vi "Initialize.vi"(8 "error in (no error)":errorcluster) -> (0 "error out":errorcluster, 3 "config":T1={"Common"={"State"=enum."Off", "Waveform Channel"="", "DataGroup"="", "Number of Samples"=0, "Timeout"=0.0, "History"=variant, "LastRequest"=timestamp(0 s since 1904-01-01), "BufferSize"=0, "OpState"=variant, "IRoutingSource"={"CorrelationId"="", "ReplyTo"=""}}, "CameraInfo"=variant(string[] [])})   [LabVIEW 2017, in "IrTestPanel.lvlib"]
uses:
  <vilib>/addons/InsightCM/Devices/Shared/Ir/IrTestPanel/IrTestPanel.lvlib
  <vilib>/addons/InsightCM/Devices/Shared/Ir/IrTestPanel/controls/config.ctl
  <vilib>/addons/InsightCM/Devices/Shared/Common/TestPanel/controls/Configuration.ctl
  <vilib>/addons/InsightCM/Devices/Shared/Common/TestPanel/controls/State.ctl
  <vilib>/addons/InsightCM/MessageBus/Base/controls/IRoutingSource.ctl
  <vilib>/addons/InsightCM/MessageBus/Base/controls/TestPanelTimeSeries.ctl
  <vilib>/addons/InsightCM/MessageBus/Base/controls/TestPanelValue.ctl
  <vilib>/addons/InsightCM/Utilities/PropertyHelpers/PropertyHelpers.lvlib
  <vilib>/addons/InsightCM/Utilities/GlobalConfiguration/GlobalConfiguration.lvlib
  <vilib>/addons/InsightCM/Devices/Shared/Common/TestPanel/TestPanel.lvlib
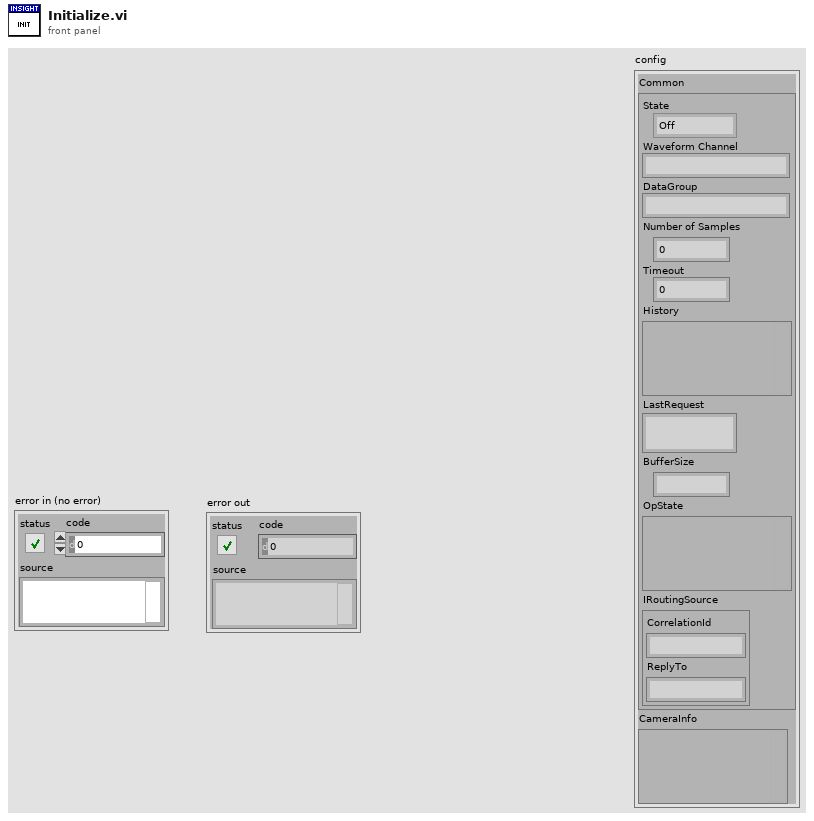
[diagram p1: front panel]
types:
  T1 = typedef "IrTestPanel.lvlib/config.ctl" = cluster{"Common":T2, "CameraInfo":variant}
  T2 = typedef "TestPanel.lvlib/Configuration.ctl" = cluster{"State":T3, "Waveform Channel":string, "DataGroup":string, "Number of Samples":i32, "Timeout":dbl, "History":variant, "LastRequest":timestamp, "BufferSize":i32, "OpState":variant, "IRoutingSource":T4}
  T3 = typedef "TestPanel.lvlib/State.ctl" = enum16{"Off", "On", "PendingValues", "PendingDataSet"}
  T4 = typedef "IRoutingSource.ctl" = cluster{"CorrelationId":string, "ReplyTo":string}
  T5 = typedef "SectionKeyValues.ctl" = cluster{"Section":string, "KeyValues":T6[]}
  T6 = typedef "KeyValuePair.ctl" = cluster{"Key":string, "Value":string}
  T7 = typedef "R2_Channel.ctl" = cluster{"Id":string, "DeviceId":string, "Name":string, "ChannelType":string, "HardwareKey":string, "HardwareChannel":string, "DataGroup":string, "Keywords":string[], "EquipmentIds":string[], "Properties":T6[], "Metrics":T8[], "AssetNodeId":string, "MeasType":string, "AssetName":string}
  T8 = typedef "Metric.ctl" = cluster{"Id":string, "Name":string, "Unit":string, "Properties":T6[], "MetricDefinitionInstanceId":string}
  T9 = typedef "AssetNode.ctl" = cluster{"Id":string, "Type":string, "Name":string, "ParentIds":string[], "State":T10, "MeasType":string, "Properties":T6[], "OperatingStates":T11[], "Metrics":T8[], "TrendAlarmRules":T14[], "References":T17[]}
  T10 = typedef "AssetState.ctl" = cluster{"Disabled":bool}
  T11 = typedef "OperatingState.ctl" = cluster{"Name":string, "Properties":T6[], "Triggers":T12[]}
  T12 = typedef "Trigger.ctl" = cluster{"Type":string, "Expression":string, "Conditions":T13[]}
  T13 = typedef "Condition.ctl" = cluster{"Source":string, "Type":string, "Operator":string, "CompareTo":string, "DwellSeconds":dbl}
  T14 = typedef "TrendAlarmRule.ctl" = cluster{"Id":string, "AssetNodeId":string, "TrendId":string, "Disabled":bool, "OperatingState":string, "Operator":string, "Hysteresis":dbl, "OnDelaySeconds":dbl, "OffDelaySeconds":dbl, "Levels":T15[], "Properties":T6[]}
  T15 = typedef "TrendAlarmLevel.ctl" = cluster{"Severity":i32, "CompareTo":dbl, "Actions":T16[]}
  T16 = typedef "AlarmAction.ctl" = cluster{"Type":string, "Props":T6[]}
  T17 = typedef "AssetNodeReference.ctl" = cluster{"NodeId":string, "Name":string}
  T18 = typedef "TestPanelTimeSeries.ctl" = cluster{"TrendPointId":string, "AssetName":string, "MetricName":string, "Unit":string, "Values":T19[]}
  T19 = typedef "TestPanelValue.ctl" = cluster{"Value":dbl, "Timestamp":i64, "Invalid":bool}
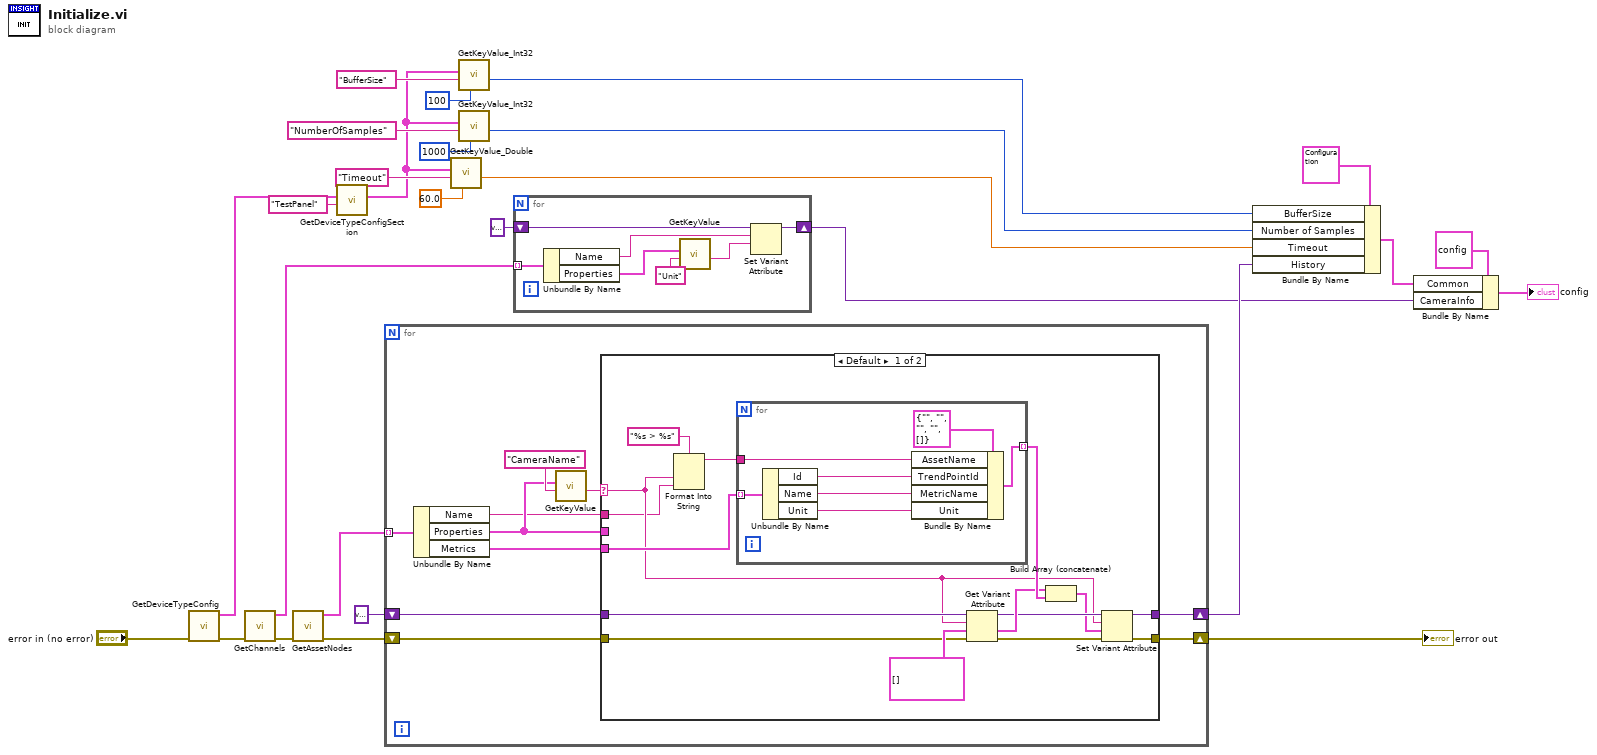
[diagram p0: block diagram]
diagram:
  n1 = call <vilib>:"GetDeviceTypeConfig.vi"("error in (no error)"="error in (no error)") -> ("error out"=w3:errorcluster, "key values"=w27:T5[])  [unwired: 8 in, 1 out]
  n2 = call <vilib>:"GetChannels.vi"("error in (no error)"=w3) -> ("error out"=w2:errorcluster, "channels"=w1:T7[])  [unwired: 8 in, 1 out]
  n3 = call <vilib>:"GetAssetNodes.vi"("error in (no error)"=w2) -> ("error out"=w12:errorcluster, "AssetNodes"=w14:T9[])  [unwired: 8 in, 1 out]
  n4 = call <vilib>:"GetDeviceTypeConfigSection.vi"("key"="TestPanel", "key values"=w27) -> ("key value pairs out"=w18:T6[])  [unwired: 8 in, 1 out]
  n5 = for {
    tunnel: w14 -> [w37] mode=indexing
    shift-right: [w29] -> w10
    shift-left: variant -> [w32]
    shift-right: [w30] -> w11
    shift-left: w12 -> [w31]
    n6 = Unbundle By Name(w37) -> ("Name"=w28:string, "Properties"=w34:T6[], "Metrics"=w36:T8[])
    n7 = call <vilib>:"GetKeyValue.vi"("key"="CameraName", "key value pairs"=w34) -> ("value"=w33:string)  [unwired: 7 in, 2 out]
    n8 = case shown="Default" w33 {
      selector: w33 -> [w43 _]
      tunnel: w36 -> [w52 _]
      tunnel: w34 -> [_ _]
      tunnel: w32 -> [w50 w61]
      tunnel: w31 -> [w49 w60]
      tunnel: [w40 w60] -> w30
      tunnel: [w39 w61] -> w29
      tunnel: w28 -> [w38 _]
      frame Default {
        n9 = Format Into String(format string="%s > %s", w43, w38) -> (resulting string=w45:string)  [unwired: 2 in, 1 out]
        n10 = for {
          tunnel: w52 -> [w58] mode=indexing
          tunnel: [w56] -> w48 mode=indexing
          tunnel: w45 -> [w55]
          n11 = Unbundle By Name(w58) -> ("Id"=w57:string, "Name"=w54:string, "Unit"=w53:string)
          n12 = Bundle By Name(cluster=T18 {"TrendPointId"="", "AssetName"="", "MetricName"="", "Unit"="", "Values"=[]} ("History"), "AssetName"=w55, "TrendPointId"=w57, "MetricName"=w54, "Unit"=w53) -> (w56:T18)
        }
        n13 = Get Variant Attribute(Variant=w50, name=w43, default value (empty Variant)=T18[] [], error in=w49) -> (duplicate Variant=w44:variant, value=w47:T18[], error out=w41:errorcluster)  [unwired: 1 out]
        n14 = Build Array (concatenate)(w47, w48) -> (w42:T18[])
        n15 = Set Variant Attribute(Variant=w44, name=w43, value=w42, error in=w41) -> (Variant out=w39:variant, error out=w40:errorcluster)  [unwired: 1 out]
      }
      frame "" {
      }
    }
  }
  "error out" <- w11
  n16 = call <vilib>:"GetKeyValue_Double.vi"("default"=60.0, "key"="Timeout", "key value pairs"=w18) -> ("value"=w21:dbl)  [unwired: 6 in, 2 out]
  n17 = call <vilib>:"GetKeyValue_Int32.vi"("default"=100, "key"="BufferSize", "key value pairs"=w18) -> ("value"=w16:i32)  [unwired: 6 in, 2 out]
  n18 = call <vilib>:"GetKeyValue_Int32.vi"("default"=1000, "key"="NumberOfSamples", "key value pairs"=w18) -> ("value"=w20:i32)  [unwired: 6 in, 2 out]
  n19 = for {
    tunnel: w1 -> [w68] mode=indexing
    shift-right: [w66] -> w4
    shift-left: variant -> [w67]
    n20 = Unbundle By Name(w68) -> ("Name"=w65:string, "Properties"=w64:T6[])
    n21 = call <vilib>:"GetKeyValue.vi"("key"="Unit", "key value pairs"=w64) -> ("value"=w62:string)  [unwired: 7 in, 2 out]
    n22 = Set Variant Attribute(Variant=w67, name=w65, value=w62) -> (Variant out=w66:variant)  [unwired: 1 in, 2 out]
  }
  n23 = Bundle By Name(cluster=T2 {"State"=enum."Off", "Waveform Channel"="", "DataGroup"="", "Number of Samples"=0, "Timeout"=0.0, "History"=variant, "LastRequest"=timestamp(0 s since 1904-01-01), "BufferSize"=0, "OpState"=variant, "IRoutingSource"={"CorrelationId"="", "ReplyTo"=""}} ("Common"), "BufferSize"=w16, "Number of Samples"=w20, "Timeout"=w21, "History"=w10) -> (w7:T2)
  n24 = Bundle By Name(cluster=T1 {"Common"={"State"=enum."Off", "Waveform Channel"="", "DataGroup"="", "Number of Samples"=0, "Timeout"=0.0, "History"=variant, "LastRequest"=timestamp(0 s since 1904-01-01), "BufferSize"=0, "OpState"=variant, "IRoutingSource"={"CorrelationId"="", "ReplyTo"=""}}, "CameraInfo"=variant(string[] [])} ("config"), "Common"=w7, "CameraInfo"=w4) -> (→"config":T1)
